vi "Cross Power (CDB).vi"(2 "Y":cdb[](array[numeric]), 3 "X":cdb[](array[numeric])) -> (0 "error":i32, 1 "Sxy":cdb[](array[numeric]))   [LabVIEW 2010, in "NI_AALPro.lvlib"]
doc: "Computes the cross power spectrum, <B>Sxy</B>, of the input signals <B>X</B> and <B>Y</B>. Wire data to the <B>X</B> input to determine the polymorphic instance to use or manually select the instance."
uses:
  NI_AALPro.lvlib
  lvanlys.dll
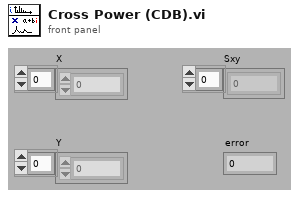
[diagram p1: front panel]
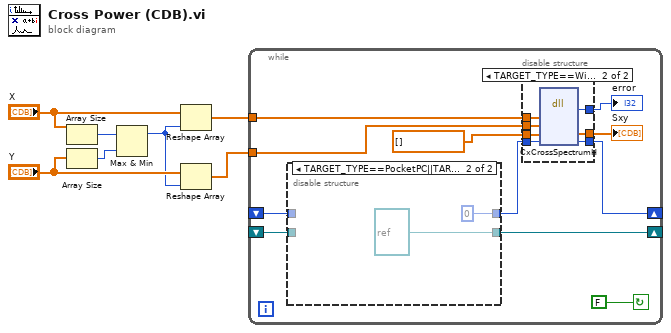
[diagram p0: block diagram]
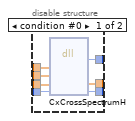
[diagram p2: hidden frame]
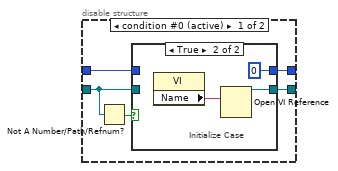
[diagram p3: hidden frame]
diagram:
  n1 = Array Size(array="X") -> (size(s)=w3:i32)
  n2 = Array Size(array="Y") -> (size(s)=w2:i32)
  n3 = Max & Min(x=w3, y=w2) -> (max(x,y)=w1:i32)  [unwired: 1 out]
  n4 = Reshape Array("X", w1) -> (w4:cdb[])
  n5 = Reshape Array("Y", w1) -> (w5:cdb[])
  n6 = while {
    tunnel: w5 -> [w15]
    shift-left: _ -> [w12]
    shift-right: [w14] -> _
    tunnel: w4 -> [w18]
    shift-right: [w10] -> _
    shift-left: _ -> [w11]
    stop <- FALSE continue-if-true
    n7 = disable-structure shown="TARGET_TYPE==PocketPC||TARGET_TYPE==PalmOS||TARGET_TYPE==FPGA||TARGET_TYPE==Embedded" {
      disable-tunnel: w11 -> [w35 _]
      disable-tunnel: [w36 refnum<vi> refnum ("VI Refnum")] -> w10
      disable-tunnel: w12 -> [w34 _]
      disable-tunnel: [w33 0 ("t")] -> w13
      frame condition #0 (active) {
        n8 = Not A Number/Path/Refnum?(number/path/refnum=w35) -> (NaN/Path/Refnum?=w37:bool)
        n9 = case shown="True" w37 {
          tunnel: [w39 w41] -> w36
          tunnel: w35 -> [w39 _]
          tunnel: w34 -> [w38 _]
          tunnel: [w38 0 ("error")] -> w33
          frame False {
          }
          frame True {
            # "Initialize Case"
            n10 = property class="VI"() -> ("Name"=w40:string)  [unwired: 2 in, 2 out]
            n11 = Open VI Reference(vi path=w40) -> (vi reference=w41:refnum<vi>)  [unwired: 5 in, 1 out]
          }
        }
      }
      frame condition #1 {
      }
    }
    n12 = disable-structure shown="TARGET_TYPE==Windows||TARGET_TYPE==Mac||TARGET_TYPE==Unix" {
      disable-tunnel: w18 -> [w25 w32]
      disable-tunnel: [w24 w31] -> w17
      disable-tunnel: [w23 w30] -> w9
      disable-tunnel: w15 -> [w22 w29]
      disable-tunnel: [w21 w28] -> w14
      disable-tunnel: w13 -> [w20 w27]
      disable-tunnel: cdb[] [] ("Sxy") -> [w19 w26]
      frame condition #0 {
        n13 = dll-call lib="C:/Program Files/National Instruments/LabVIEW 2010/resource/lvanlys.dll" fn="CxCrossSpectrumH"("X"=w25, "Y"=w22, w19, "tbl"=w20) -> (w24:i32, w23:cdb[], "tbl"=w21:i32)  [unwired: 5 in, 2 out]
      }
      frame condition #1 (active) {
        n14 = dll-call lib="C:/Program Files/National Instruments/LabVIEW 2010/resource/lvanlys.dll" fn="CxCrossSpectrumH"("xH"=w32, "yH"=w29, "zH"=w26, "tbl"=w27) -> ("return type"=w31:i32, "zH"=w30:cdb[], "tbl"=w28:i64)  [unwired: 5 in, 2 out]
      }
    }
    "Sxy" <- w9
    "error" <- w17
  }
